vi "midiOutNoteOn.vi"(8 "error in":errorcluster, 9 "Velocity (0-127)":i32, 10 "Note (0-127)":i32, 11 "midi in":refnum<class "midi.lvclass">) -> (0 "error out":errorcluster, 3 "midi out":refnum<class "midi.lvclass">)   [LabVIEW 2020, in "midi.lvclass"]
uses:
  midi.lvclass
  midichannel.get.vi
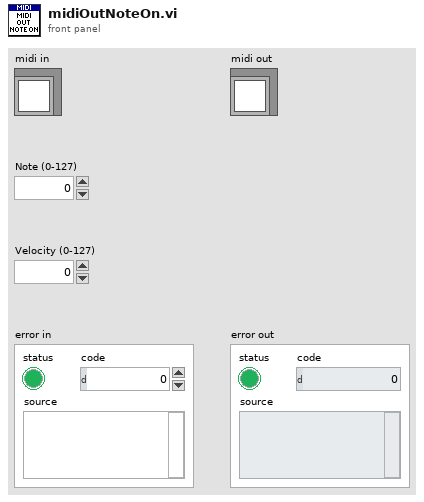
[diagram p1: front panel]
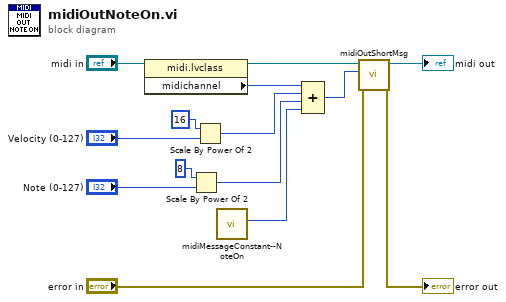
[diagram p0: block diagram]
diagram:
  n1 = property class="midi.lvclass"(reference="midi in") -> (reference out=w2:refnum<class "midi.lvclass">, "midichannel"=w1:u64)  [unwired: 1 in, 1 out]
  n2 = Scale By Power Of 2(n=8, x="Note (0-127)") -> (x*2^n=w14:i32)
  n3 = Scale By Power Of 2(n=i16 16, x="Velocity (0-127)") -> (x*2^n=w13:i32)
  n4 = call "midiMessageConstant--NoteOn.vi"() -> ("Message"=w4:u8)  [unwired: 11 in]
  n5 = Compound Arithmetic op=ADD(w1, w13, w14, w4) -> (w8:u64)
  n6 = call "midiOutShortMsg.vi"("error in"="error in", "data"=w8, "midi in"=w2) -> ("error out"=→"error out":errorcluster, "midi out"=→"midi out":refnum<class "midi.lvclass">)  [unwired: 7 in]
